vi "Actor Core.vi"(8 "error in":errorcluster, 11 "Blackstart in":refnum<class "Blackstart.lvclass">) -> (0 "error out":errorcluster, 3 "Actor out":refnum<class "Actor.lvclass">)   [LabVIEW 2018, in "Blackstart Actor.lvlib" / "Blackstart.lvclass"]
doc: "(<B>Filename</B>: Actor Framework.lvlib:Actor.lvclass:Actor Core.vi)\n\nReceives messages to the actor, reacts to them, and initiates any error handling that may shut the actor down.\n\nDescendant classes may override this VI to append parallel tasks for the actor to complete while it handles messages. Overrides use the Call Parent Method node."
uses:
  Blackstart.lvclass
  C:/Program Files (x86)/National Instruments/LabVIEW 2018/vi.lib/ActorFramework/Actor/Actor.lvclass
  C:/Users/Administrator/Desktop/LabVIEW EMS/EMS Generic Actor/EMS Generic/EMS Generic.lvclass
  C:/Users/Administrator/Desktop/LabVIEW EMS/Optimization/Startup Optimization Actor/Startup Optimization/Startup Optimization.lvclass
  C:/Users/Administrator/Desktop/LabVIEW EMS/Device Communication and Control Abstract Actor/Device Communication and Control Abstract/Device Communication and Control Abstract.lvclass
  C:/Users/Administrator/Desktop/LabVIEW EMS/Optimization/Generic Optimization Actor/Generic Optimization/Generic Optimization.lvclass
  <vilib>/ActorFramework/Actor/Actor.lvclass
  Controls/Blackstart State.ctl
  <vilib>/ORNL/CSEISMIC DDS/CSEISMIC DDS Base/Data Types/Controls/DeviceID.ctl
  <vilib>/ActorFramework/Actor/Actor.lvclass/Actor.ctl
  EMS Generic Actor/EMS Generic/EMS Generic.lvclass/EMS Generic.ctl
  <vilib>/ActorFramework/Message Enqueuer/Message Enqueuer.lvclass/Message Enqueuer.ctl
  <vilib>/ORNL/CSEISMIC DDS/CSEISMIC DDS Base/Data Types/DER_VF.ctl
  Startup Optimization Actor/Startup Optimization/Startup Optimization.lvclass/Startup Optimization.ctl
  Device Communication and Control Abstract Actor/Device Communication and Control Abstract/Device Communication and Control Abstract.lvclass/Device Communication and Control Abstract.ctl
  Device Communication and Control Abstract Actor/Device Communication and Control Abstract Messages/Set DER VF Msg/Set DER VF Msg.lvclass/Set DER VF Msg.ctl
  <vilib>/ORNL/CSEISMIC DDS/CSEISMIC DDS Base/Data Types/PCC_Transition.ctl
  Device Communication and Control Abstract Actor/Device Communication and Control Abstract Messages/Set PCC Transition Msg/Set PCC Transition Msg.lvclass/Set PCC Transition Msg.ctl
  <vilib>/ORNL/CSEISMIC DDS/CSEISMIC DDS Base/Data Types/DER_Control.ctl
  <vilib>/ORNL/CSEISMIC DDS/CSEISMIC DDS Base/Data Types/DER_setGenerationMode.ctl
  <vilib>/ORNL/CSEISMIC DDS/CSEISMIC DDS Base/Data Types/Controls/Generation Mode.ctl
  Device Communication and Control Abstract Actor/Device Communication and Control Abstract Messages/Set DER GenerationMode Msg/Set DER GenerationMode Msg.lvclass/Set DER GenerationMode Msg.ctl
  Device Communication and Control Abstract Actor/Device Communication and Control Abstract Messages/Set DER Control Msg/Set DER Control Msg.lvclass/Set DER Control Msg.ctl
  <vilib>/ORNL/CSEISMIC DDS/CSEISMIC DDS Base/Data Types/Relay_Control.ctl
  Device Communication and Control Abstract Actor/Device Communication and Control Abstract Messages/Set Relay Control Msg/Set Relay Control Msg.lvclass/Set Relay Control Msg.ctl
  <vilib>/ORNL/CSEISMIC DDS/CSEISMIC DDS Base/Data Types/Load_Control.ctl
  Device Communication and Control Abstract Actor/Device Communication and Control Abstract Messages/Set Load Control Msg/Set Load Control Msg.lvclass/Set Load Control Msg.ctl
  <vilib>/ActorFramework/Message Enqueuer/Init from Existing Queue.vi
  <vilib>/ActorFramework/Message Enqueuer/Enqueue.vi
  Device Communication and Control Abstract Actor/Device Communication and Control Abstract Messages/Set DER VF Msg/Send Set DER VF.vi
  Device Communication and Control Abstract Actor/Device Communication and Control Abstract Messages/Set PCC Transition Msg/Send Set PCC Transition.vi
  Device Communication and Control Abstract Actor/Device Communication and Control Abstract Messages/Set DER GenerationMode Msg/Send Set DER GenerationMode.vi
  Device Communication and Control Abstract Actor/Device Communication and Control Abstract Messages/Set DER Control Msg/Send Set DER Control.vi
  Device Communication and Control Abstract Actor/Device Communication and Control Abstract Messages/Set Relay Control Msg/Send Set Relay Control.vi
  Device Communication and Control Abstract Actor/Device Communication and Control Abstract Messages/Set Load Control Msg/Send Set Load Control.vi
  Device Communication and Control Abstract Actor/Device Communication and Control Abstract/Device Communication and Control Abstract.lvclass
  Device Communication and Control Abstract Actor/Device Communication and Control Abstract Messages/Set DER VF Msg/Set DER VF Msg.lvclass
  C:/Program Files (x86)/National Instruments/LabVIEW 2018/vi.lib/ActorFramework/Message/Message.lvclass
  Device Communication and Control Abstract Actor/Device Communication and Control Abstract Messages/Set PCC Transition Msg/Set PCC Transition Msg.lvclass
  Device Communication and Control Abstract Actor/Device Communication and Control Abstract Messages/Set DER GenerationMode Msg/Set DER GenerationMode Msg.lvclass
  Device Communication and Control Abstract Actor/Device Communication and Control Abstract Messages/Set DER Control Msg/Set DER Control Msg.lvclass
  Device Communication and Control Abstract Actor/Device Communication and Control Abstract Messages/Set Relay Control Msg/Set Relay Control Msg.lvclass
  Device Communication and Control Abstract Actor/Device Communication and Control Abstract Messages/Set Load Control Msg/Set Load Control Msg.lvclass
  <vilib>/ActorFramework/Stop Msg/Stop Msg.lvclass
  <vilib>/ActorFramework/Message Priority Queue/Priority Enqueue.vi
  Startup Optimization Actor/Startup Optimization/Startup Optimization.lvclass
  <vilib>/ActorFramework/Message Enqueuer/Message Enqueuer.lvclass
  <vilib>/ORNL/CSEISMIC DDS/CSEISMIC DDS Base/CSEISMIC DDS.lvclass
  Utilities/Status Messaging.llb/Status Messaging.lvlib
  EMS Generic Actor/EMS Generic/EMS Generic.lvclass
  Generic Optimization Actor/Generic Optimization/Generic Optimization.lvclass
panel:
  out "Devices":string[](array[string])
  in  "Ignore missing devices?":bool
  out "Status":T1
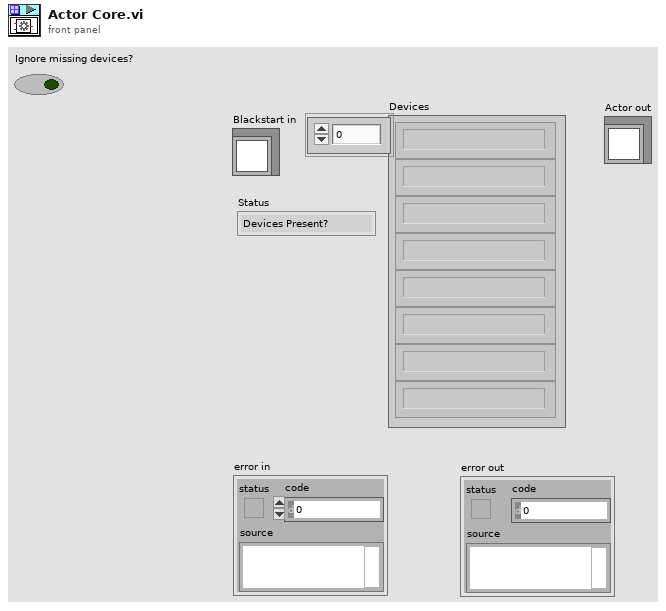
[diagram p1: front panel]
types:
  T1 = typedef "Blackstart Actor.lvlib/Blackstart.lvclass/Blackstart State.ctl" = enum16{"Devices Present?", "Group Devices", "Set VF Device", "Island", "Activate VF Device", "Close Relays", "Activate Loads", "Activate DERs", "Success", "Failure"}
  T2 = typedef "CSEISMIC DDS.lvlib/CSEISMIC DDS.lvclass/DeviceID.ctl" = string
  T3 = enum32{"Invalid", "Standard", "Closed", "Hidden", "Minimized", "Maximized"}
  T4 = typedef "CSEISMIC DDS.lvlib/CSEISMIC DDS.lvclass/DER_VF.ctl" = cluster{"DeviceID":T2}
  T5 = typedef "CSEISMIC DDS.lvlib/CSEISMIC DDS.lvclass/DER_setGenerationMode.ctl" = cluster{"DeviceID":T2, "Mode":T6}
  T6 = typedef "CSEISMIC DDS.lvlib/CSEISMIC DDS.lvclass/Generation Mode.ctl" = enum32{"Invalid", "PQ", "Droop", "PV", "PF", "VF"}
  T7 = typedef "CSEISMIC DDS.lvlib/CSEISMIC DDS.lvclass/DER_Control.ctl" = cluster{"DeviceID":T2, "Activate":bool, "Deactivate":bool}
  T8 = typedef "EMS Generic Actor.lvlib/EMS Generic.lvclass/Global Configuration.ctl" = cluster{"Microgrid ID":u8, "VF Device ID":T2, "Ongrid VF Priority":T2[], "Offgrid VF Priority":T2[], "AutoSwap Offgrid VF":u32, "AutoSwap Offgrid VF Delay (sec)":dbl, "AutoSwap Resynch VF":u32, "PCC Device ID":T2, "Device ID Array":T2[], "Nominal Voltage":dbl, "Nominal Frequency":dbl, "Resynch Timeout (sec)":dbl, "Island VF Activate Timeout (sec)":dbl, "Island PCC Target Power (kW)":dbl, "Island PCC Target Power Timeout (sec)":dbl, "Island Grid Settle Time (sec)":dbl, "Island PCC Failure Timeout (sec)":dbl, "Activation Devices Present Timeout (sec)":dbl, "Activation Devices Activated Timeout (sec)":dbl, "Blackstart VF GenMode Wait (sec)":dbl, "Blackstart VF DERCtrl Wait (sec)":dbl, "Blackstart Success Wait (sec)":dbl, "OnGrid Optimization Delay (sec)":dbl, "OffGrid Optimization Delay (sec)":dbl, "Resynch Frequency (Hz)":dbl, "Optimization Path":string}
  T9 = typedef "CSEISMIC DDS.lvlib/CSEISMIC DDS.lvclass/PCC_Transition.ctl" = cluster{"DeviceID":T2, "Island":bool, "Resynchronize":bool}
  T10 = typedef "CSEISMIC DDS.lvlib/CSEISMIC DDS.lvclass/IED_Status.ctl" = cluster{"DeviceID":T2, "Timestamp":T11, "MicrogridID":u8, "Active":bool, "Inactive":bool, "Error":i32, "Fault":bool, "ErrorString":string}
  T11 = typedef "CSEISMIC DDS.lvlib/CSEISMIC DDS.lvclass/Timestamp.ctl" = cluster{"Seconds":u64, "Remainder":u64}
  T12 = typedef "CSEISMIC DDS.lvlib/CSEISMIC DDS.lvclass/Relay_Control.ctl" = cluster{"DeviceID":T2, "Activate":bool, "Deactivate":bool}
  T13 = typedef "CSEISMIC DDS.lvlib/CSEISMIC DDS.lvclass/Load_Control.ctl" = cluster{"DeviceID":T2, "Activate":bool, "Deactivate":bool}
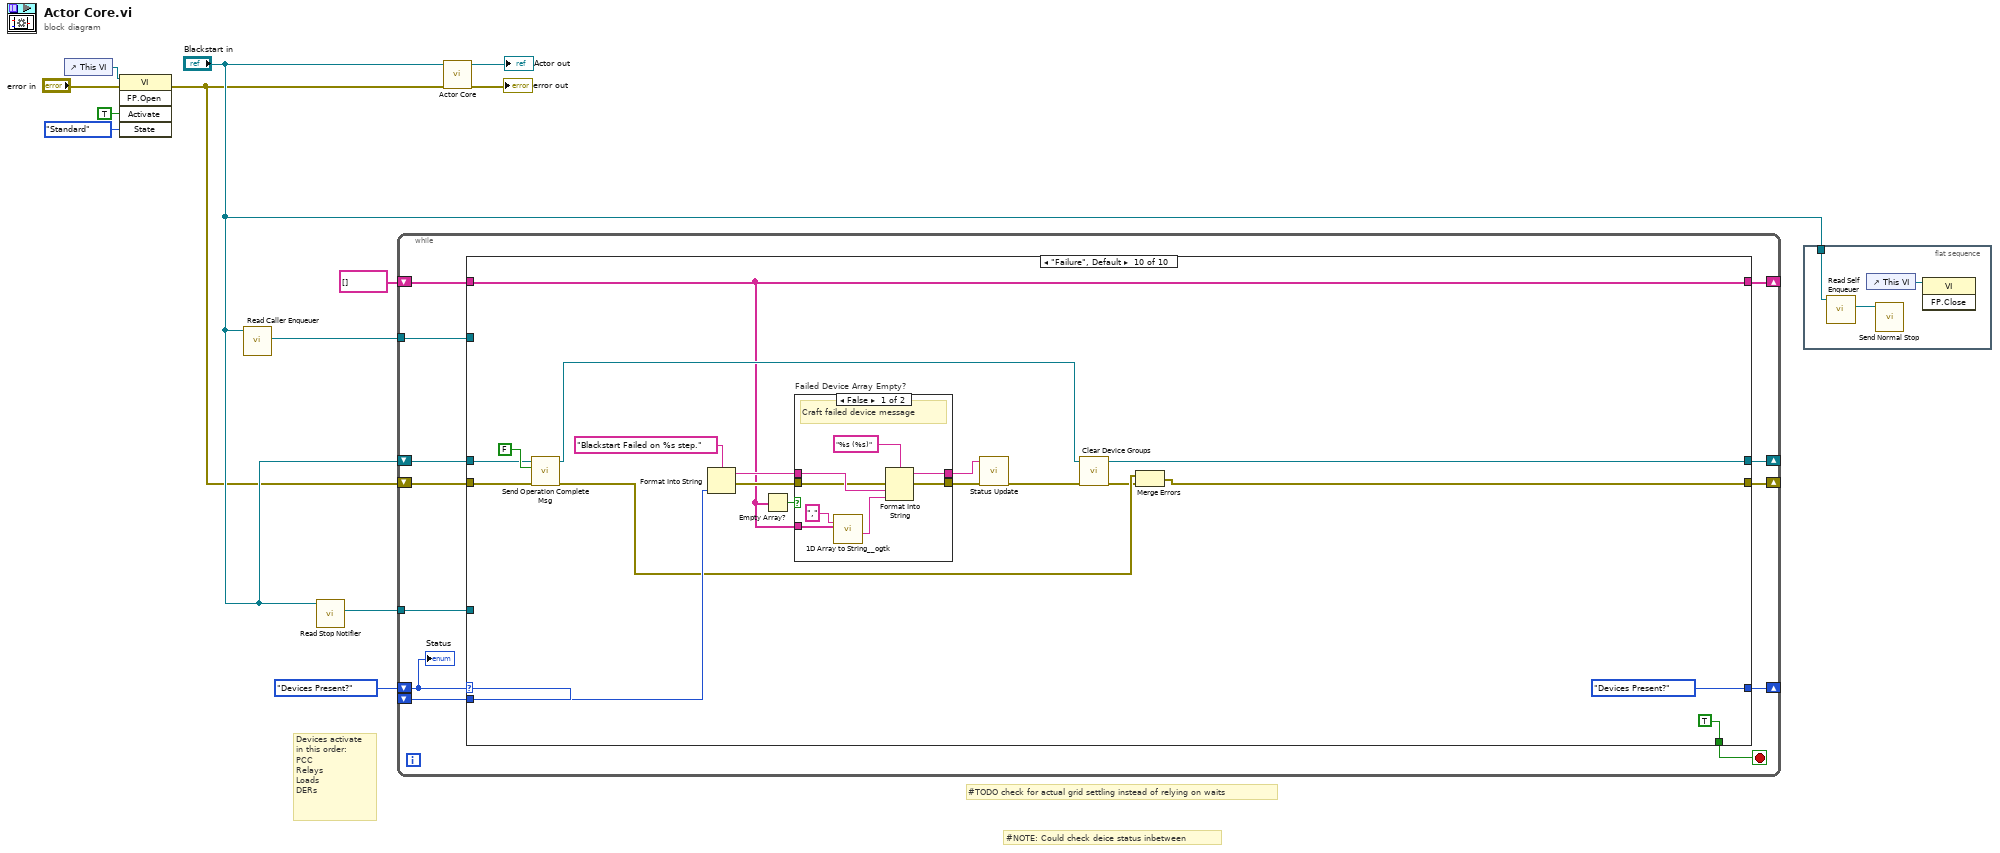
[diagram p0: block diagram]
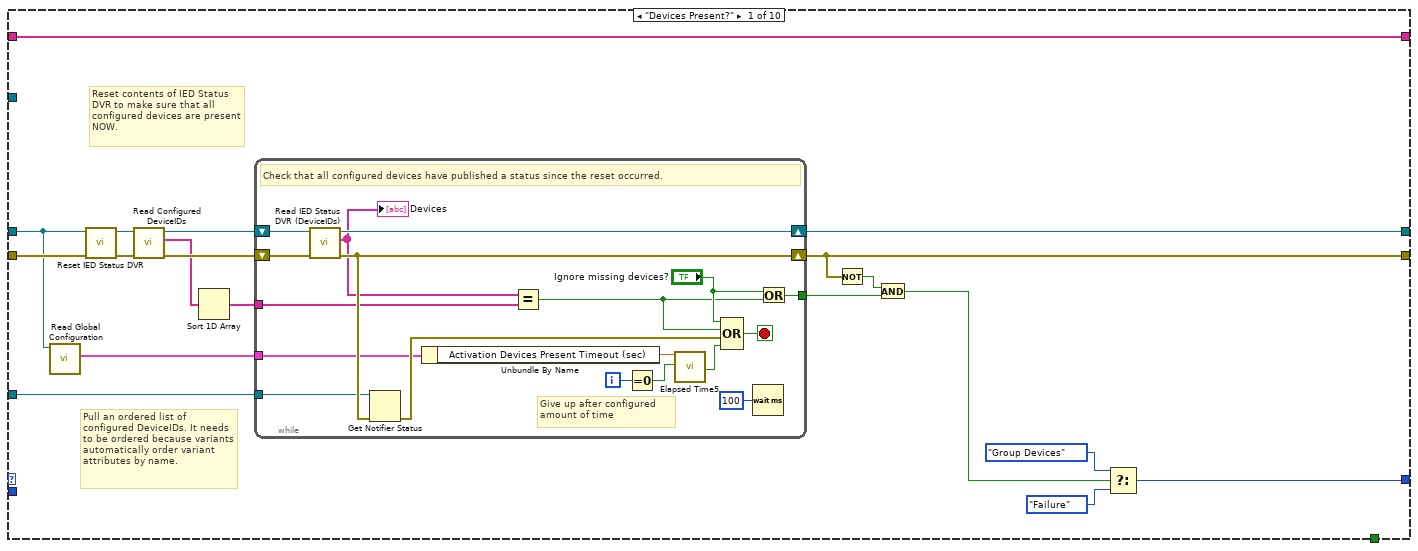
[diagram p2: hidden frame]
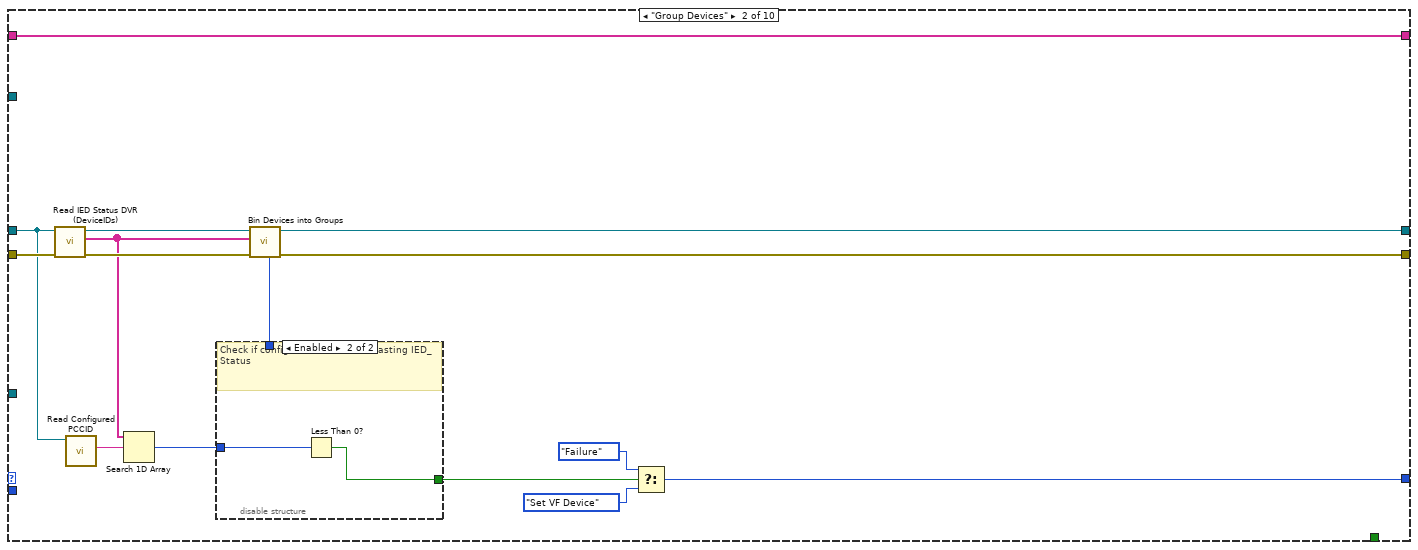
[diagram p3: hidden frame]
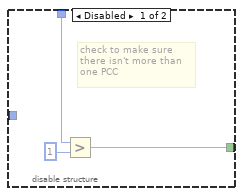
[diagram p4: hidden frame]
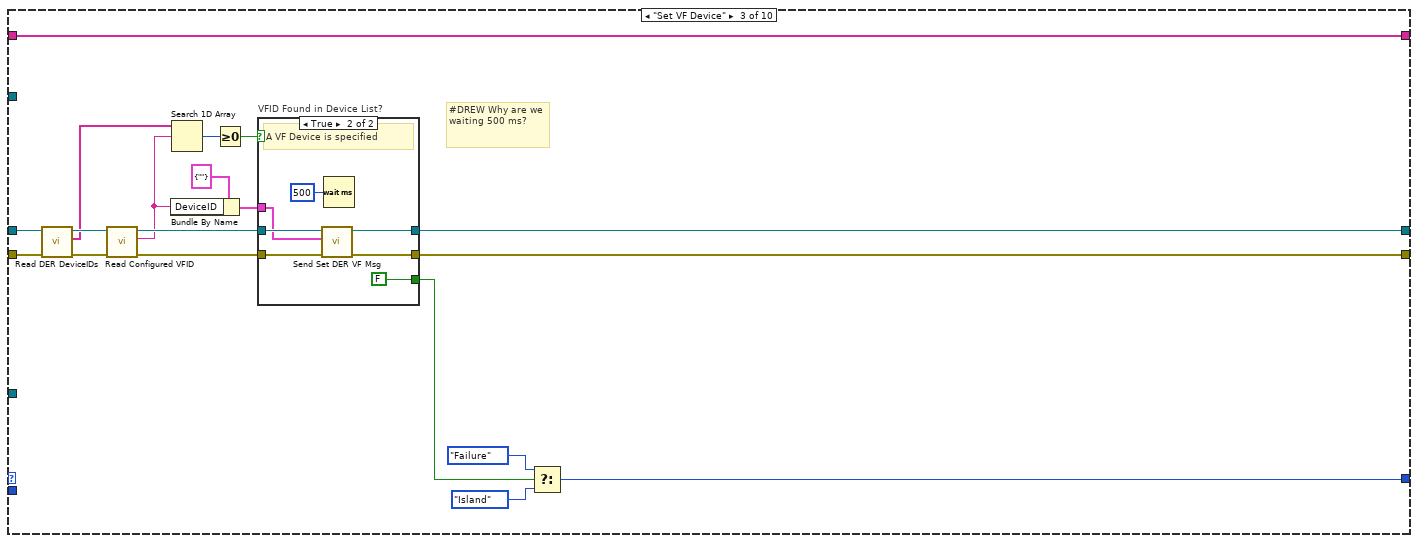
[diagram p5: hidden frame]
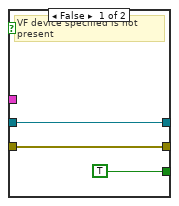
[diagram p6: hidden frame]
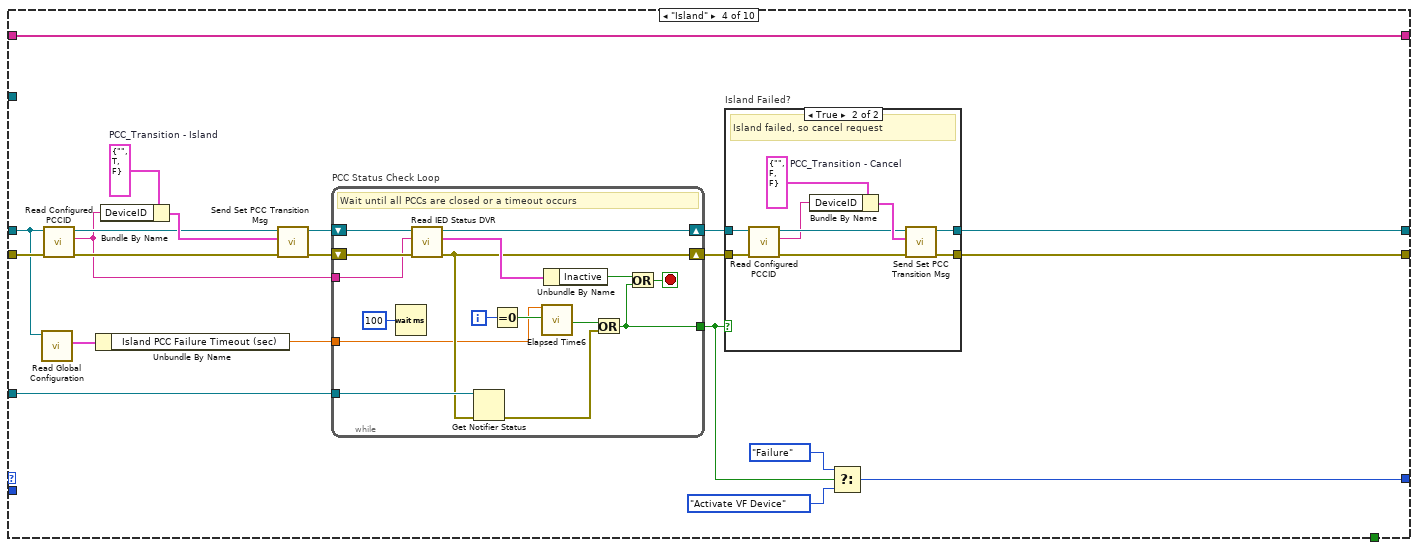
[diagram p7: hidden frame]
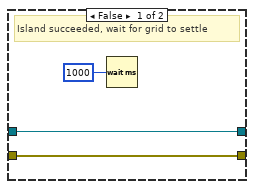
[diagram p8: hidden frame]
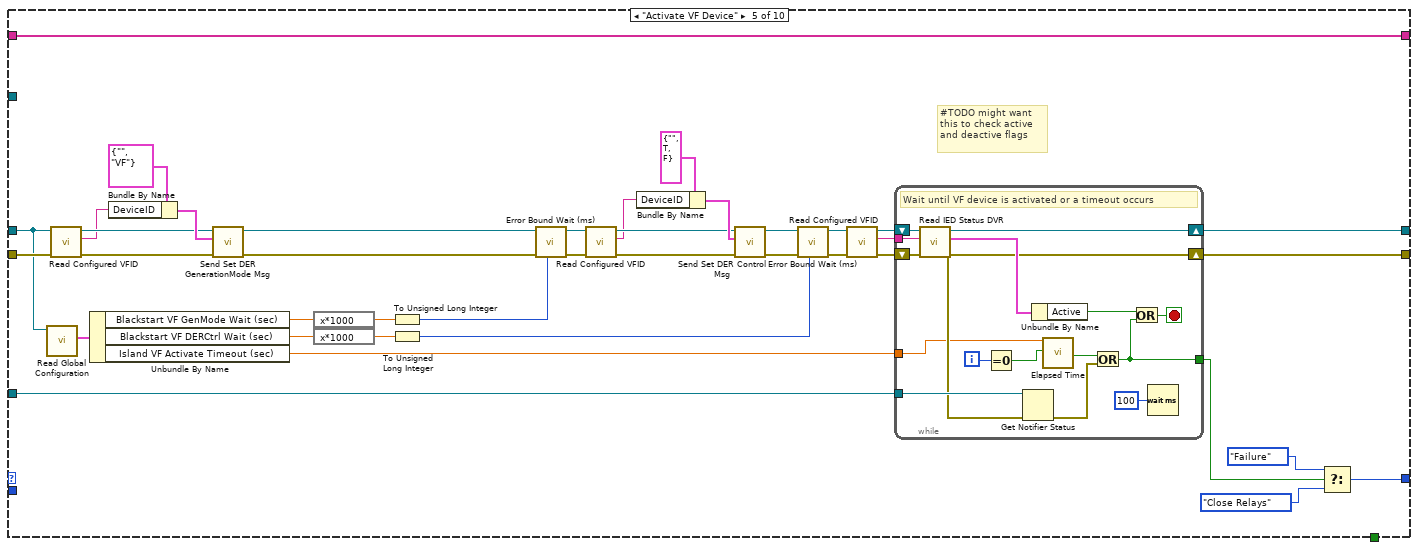
[diagram p9: hidden frame]
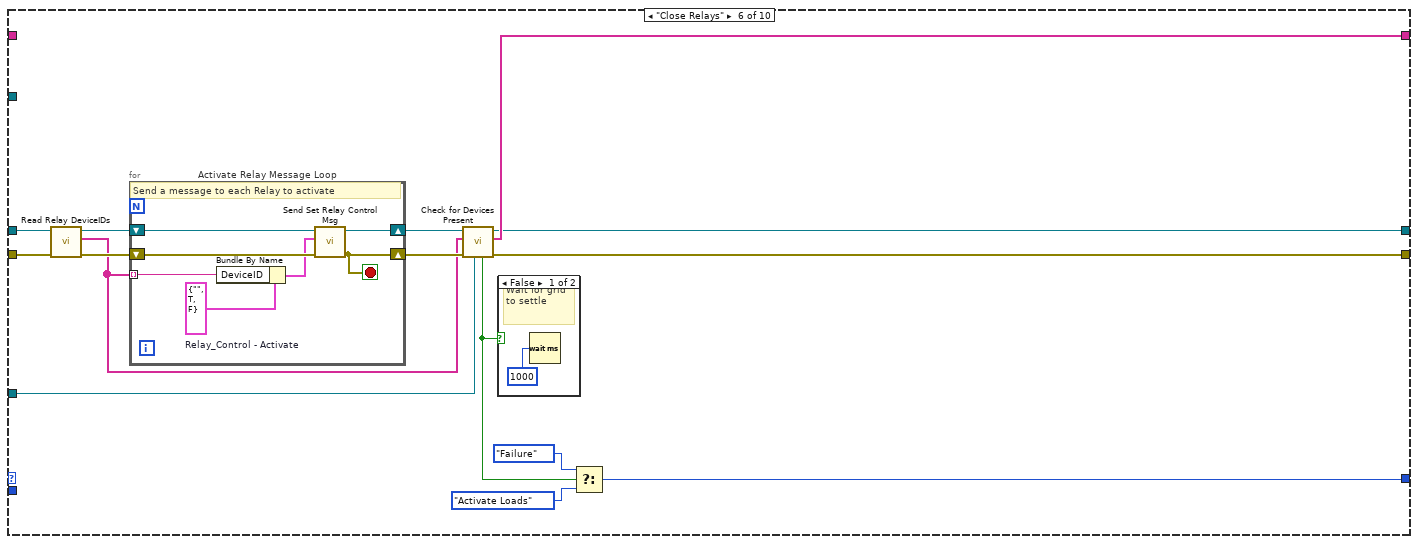
[diagram p10: hidden frame]
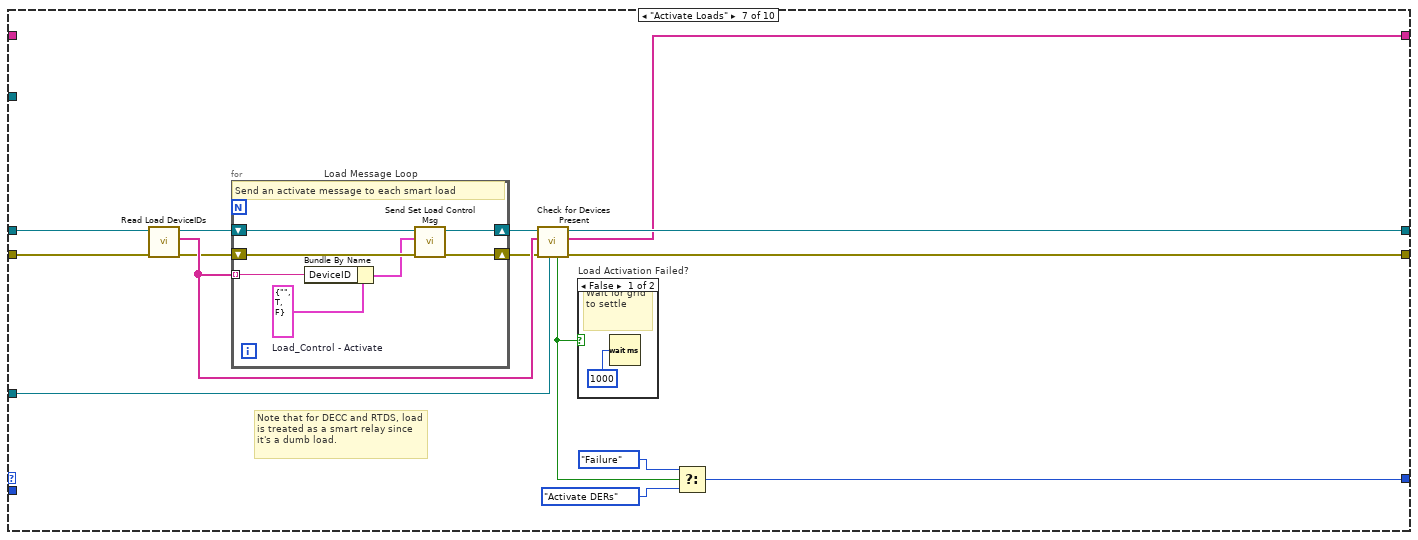
[diagram p12: hidden frame]
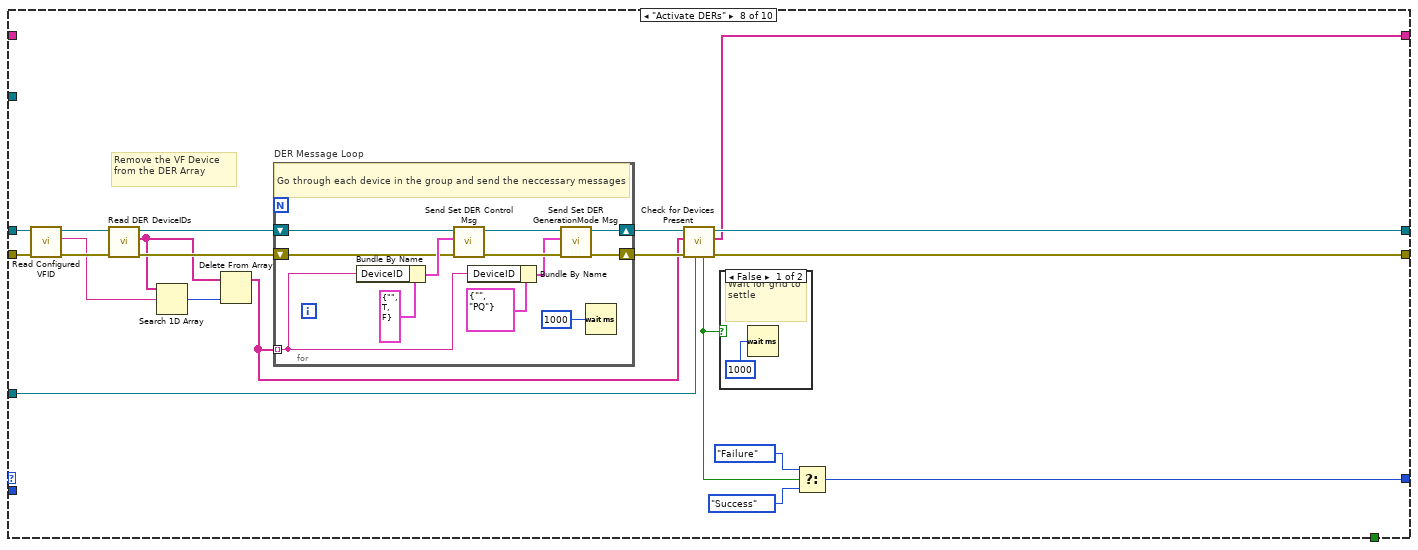
[diagram p14: hidden frame]
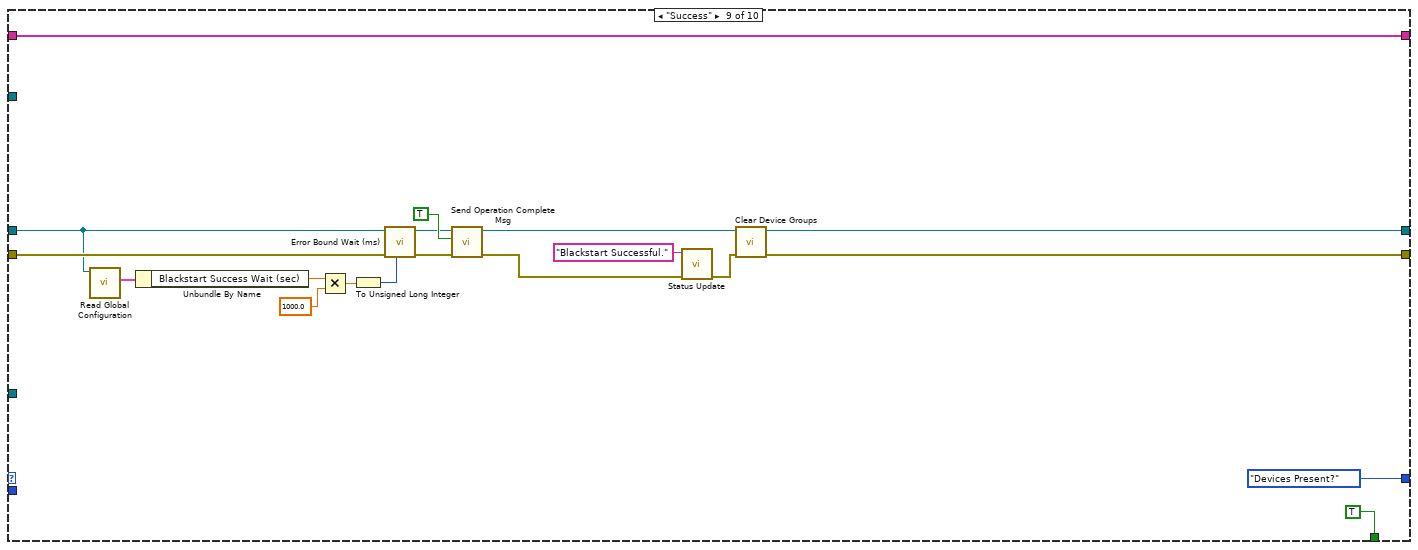
[diagram p16: hidden frame]
diagram:
  w2 = Blackstart_State."Devices Present?"
  # "#TODO check for actual grid settling instead of relying on waits"
  # "Devices activate in this order:\nPCC\nRelays\nLoads\nDERs"
  # "#NOTE: Could check deice status inbetween"
  n1 = control-ref of="This VI"() -> (w7:refnum<vi>)
  n2 = invoke class="VI" method="FP.Open"(reference=w7, error in="error in", "Activate"=TRUE ("Activate?"), "State"=T3."Standard") -> (error out=w4:errorcluster)  [unwired: 1 in, 4 out]
  n3 = call <vilib>:"Read Caller Enqueuer.vi"("Actor"="Blackstart in") -> ("Caller Enqueuer"=w10:refnum<class "Message Enqueuer.lvclass">)  [unwired: 10 in]
  n4 = call "Read Stop Notifier.vi"("EMS Generic in"="Blackstart in") -> ("stop"=w1:refnum<notifier>)  [unwired: 9 in, 1 out]
  n5 = while {
    shift-right: [w23] -> _
    shift-left: w2 -> [w24]
    tunnel: w10 -> [w22]
    shift-left: w2 -> [w19]
    tunnel: w1 -> [w18]
    shift-right: [w17] -> _
    shift-left: T2[] [] -> [w16]
    shift-right: [w14] -> _
    shift-left: "Blackstart in" -> [w21]
    shift-right: [w13] -> _
    shift-left: w4 -> [w15]
    stop <- w20 stop-if-true
    n6 = case shown="\"Failure\", Default" w24 {
      tunnel: [w42 w76 w98 w118 w195 w225 w248 w276 Blackstart_State."Devices Present?" Blackstart_State."Devices Present?"] -> w23
      tunnel: w22 -> [_ _ _ _ _ _ _ _ _ _]
      tunnel: w21 -> [w26 w64 w88 w113 w168 w224 w242 w268 w297 w317]
      tunnel: [_ _ _ _ _ _ _ _ TRUE TRUE] -> w20
      tunnel: w19 -> [_ _ _ _ _ _ _ _ _ w313]
      tunnel: w18 -> [w31 _ _ w124 w192 w218 w240 w264 _ _]
      tunnel: [w40 w75 w97 w131 w193 w216 w236 w261 w307 w314] -> w17
      tunnel: w16 -> [w40 w75 w97 w131 w193 _ _ _ w307 w314]
      tunnel: w15 -> [w30 w72 w86 w116 w186 w223 w241 w269 w306 w316]
      tunnel: [w29 w69 w90 w123 w170 w215 w239 w262 w301 w315] -> w14
      tunnel: [w28 w67 w91 w122 w169 w214 w238 w259 w300 w310] -> w13
      frame "Devices Present?" {
        # "Pull an ordered list of configured DeviceIDs. It needs to be ordered because variants automatically order variant attributes by name."
        # "Reset contents of IED Status DVR to make sure that all configured devices are present NOW."
        n7 = call "Read Global Configuration.vi"("EMS Generic in"=w26) -> ("Global Configuration"=w25:T8)  [unwired: 8 in, 2 out]
        n8 = call "Reset IED Status DVR.vi"("error in"=w30, "SCADA in"=w26) -> ("error out"=w38:errorcluster, "dup SCADA out"=w37:refnum<class "Blackstart.lvclass">)  [unwired: 8 in]
        n9 = call "Read Configured DeviceIDs.vi"("error in"=w38, "EMS Generic in"=w37) -> ("error out"=w34:errorcluster, "DeviceIDs"=w32:T2[], "EMS Generic out"=w39:refnum<class "Blackstart.lvclass">)  [unwired: 7 in]
        n10 = Sort 1D Array(array=w32) -> (sorted array=w33:T2[])
        n11 = while {
          tunnel: w33 -> [w59]
          shift-right: [w61] -> w28
          shift-left: w34 -> [w49]
          tunnel: [w54] -> w35
          tunnel: w31 -> [w58]
          shift-right: [w47] -> w29
          shift-left: w39 -> [w48]
          tunnel: w25 -> [w45]
          i -> [w51]
          stop <- w53 stop-if-true
          # "Give up after configured amount of time"
          # "Check that all configured devices have published a status since the reset occurred."
          n12 = call "Read IED Status DVR (DeviceIDs).vi"("error in"=w49, "EMS Generic in"=w48) -> ("error out"=w61:errorcluster, "DeviceID Array"=w46:T2[], "EMS Generic out"=w47:refnum<class "Blackstart.lvclass">)  [unwired: 7 in]
          "Devices" <- w46
          n13 = Get Notifier Status(notifier=w58, error in (no error)=w61) -> (error out=w57:errorcluster)  [unwired: 4 out]
          n14 = Unbundle By Name(w45) -> ("Activation Devices Present Timeout (sec)"=w44:dbl)
          n15 = Equal?(x=w46, y=w59) -> (x = y?=w55:bool)
          n16 = Equal To 0?(x=w51) -> (x = 0?=w50:bool)
          n17 = call "Elapsed Time5"("Time Target (s)"=w44, "Reset"=w50) -> ("Time has Elapsed"=w52:bool)  [unwired: 10 in, 7 out]
          n18 = Compound Arithmetic op=OR("Ignore missing devices?", w55, w57, w52) -> (w53:bool)
          n19 = Wait (ms)(milliseconds to wait=u32 100) -> ()  [unwired: 1 out]
          n20 = Or(x="Ignore missing devices?", y=w55) -> (x .or. y?=w54:bool)
        }
        n21 = Not(x=w28) -> (.not. x?=w36:bool)
        n22 = And(x=w36, y=w35) -> (x .and. y?=w27:bool)
        n23 = Select(t=Blackstart_State."Group Devices", s=w27, f=Blackstart_State."Failure") -> (s? t:f=w42:T1)
      }
      frame "Group Devices" {
        n24 = call "Read IED Status DVR (DeviceIDs).vi"("error in"=w72, "EMS Generic in"=w64) -> ("error out"=w68:errorcluster, "DeviceID Array"=w63:T2[], "EMS Generic out"=w70:refnum<class "Blackstart.lvclass">)  [unwired: 7 in]
        n25 = call "Read Configured PCCID.vi"("EMS Generic in"=w64) -> ("PCCID"=w65:T2)  [unwired: 8 in, 2 out]
        n26 = Search 1D Array(1D array=w63, element=w65) -> (index of element=w62:i32)  [unwired: 1 in]
        n27 = call "Bin Devices into Groups.vi"("error in (no error)"=w68, "DeviceID Array"=w63, "Startup Optimization in"=w70) -> ("error out"=w67:errorcluster, "Startup Optimization out"=w69:refnum<class "Blackstart.lvclass">, "Number of PCCs"=w66:i16)  [unwired: 6 in]
        n28 = disable-structure shown="Enabled" {
          disable-tunnel: [w78 w80] -> w71
          disable-tunnel: w66 -> [w77 _]
          disable-tunnel: w62 -> [_ w81]
          frame Disabled {
            # "check to make sure there isn't more than one PCC"
            n29 = Greater?(x=w77, y=i16 1) -> (0:w78:bool)
          }
          frame Enabled {
            # "Check if configured PCC is broadcasting IED_Status"
            n30 = Less Than 0?(x=w81) -> (x < 0?=w80:bool)
          }
        }
        n31 = Select(t=Blackstart_State."Failure", s=w71, f=Blackstart_State."Set VF Device") -> (s? t:f=w76:T1)
      }
      frame "Set VF Device" {
        # "#DREW Why are we waiting 500 ms?"
        n32 = call "Read DER DeviceIDs.vi"("error in"=w86, "Startup Optimization in"=w88) -> ("error out"=w85:errorcluster, "DERs"=w84:T2[], "Startup Optimization out"=w87:refnum<class "Blackstart.lvclass">)  [unwired: 7 in]
        n33 = call "Read Configured VFID.vi"("error in"=w85, "EMS Generic in"=w87) -> ("error out"=w96:errorcluster, "VFID"=w94:T2, "EMS Generic out"=w95:refnum<class "Blackstart.lvclass">)  [unwired: 7 in]
        n34 = Bundle By Name(cluster=T4 {"DeviceID"=""} ("DER_VF"), "DeviceID"=w94) -> (w93:T4)
        n35 = Search 1D Array(1D array=w84, element=w94) -> (index of element=w83:i32)  [unwired: 1 in]
        n36 = Greater Or Equal To 0?(x=w83) -> (x >= 0?=w82:bool)
        n37 = case "VFID Found in Device List?" shown="True" w82 {
          tunnel: [TRUE FALSE] -> w89
          tunnel: w93 -> [_ w107]
          tunnel: w95 -> [w102 w108]
          tunnel: [w102 w106] -> w90
          tunnel: w96 -> [w101 w105]
          tunnel: [w101 w104] -> w91
          frame False {
            # "VF device specified is not present"
          }
          frame True {
            # "A VF Device is specified"
            n38 = call "Send Set DER VF Msg.vi"("error in"=w105, "DER_VF"=w107, "SCADA Sub Abstract in"=w108) -> ("error out"=w104:errorcluster, "dup SCADA Sub Abstract"=w106:refnum<class "Blackstart.lvclass">)  [unwired: 7 in]
            n39 = Wait (ms)(milliseconds to wait=u32 500) -> ()  [unwired: 1 out]
          }
        }
        n40 = Select(t=Blackstart_State."Failure", s=w89, f=Blackstart_State."Island") -> (s? t:f=w98:T1)
      }
      frame "Island" {
        w125 = T9 {"DeviceID"="", "Island"=TRUE, "Resynchronize"=FALSE}  # PCC_Transition - Island
        n41 = call "Read Global Configuration.vi"("EMS Generic in"=w113) -> ("Global Configuration"=w117:T8)  [unwired: 8 in, 2 out]
        n42 = call "Read Configured PCCID.vi"("error in"=w116, "EMS Generic in"=w113) -> ("error out"=w114:errorcluster, "PCCID"=w111:T2, "EMS Generic out"=w115:refnum<class "Blackstart.lvclass">)  [unwired: 7 in]
        n43 = Unbundle By Name(w117) -> ("Island PCC Failure Timeout (sec)"=w112:dbl)
        n44 = Bundle By Name(cluster=w125, "DeviceID"=w111) -> (w130:T9)
        n45 = call "Send Set PCC Transition Msg.vi"("error in"=w114, "PCC_Transition"=w130, "SCADA Sub Abstract in"=w115) -> ("error out"=w128:errorcluster, "dup SCADA Sub Abstract"=w129:refnum<class "Blackstart.lvclass">)  [unwired: 7 in]
        n46 = while "PCC Status Check Loop" {
          tunnel: [w157] -> w119
          tunnel: w124 -> [w156]
          shift-right: [w148] -> w126
          shift-left: w128 -> [w145]
          shift-right: [w149] -> w127
          shift-left: w129 -> [w146]
          tunnel: w112 -> [w147]
          tunnel: w111 -> [w144]
          i -> [w155]
          stop <- w158 stop-if-true
          # "Wait until all PCCs are closed or a timeout occurs"
          n47 = Wait (ms)(milliseconds to wait=u32 100) -> ()  [unwired: 1 out]
          n48 = call "Read IED Status DVR.vi"("error in"=w145, "DeviceID"=w144, "EMS Generic in"=w146) -> ("error out"=w148:errorcluster, "IED_Status"=w152:T10, "EMS Generic out"=w149:refnum<class "Blackstart.lvclass">)  [unwired: 5 in, 1 out]
          n49 = Get Notifier Status(notifier=w156, error in (no error)=w148) -> (error out=w150:errorcluster)  [unwired: 4 out]
          n50 = Equal To 0?(x=w155) -> (x = 0?=w154:bool)
          n51 = call "Elapsed Time6"("Time Target (s)"=w147, "Reset"=w154) -> ("Time has Elapsed"=w151:bool)  [unwired: 10 in, 7 out]
          n52 = Unbundle By Name(w152) -> ("Inactive"=w159:bool)
          n53 = Or(x=w151, y=w150) -> (x .or. y?=w157:bool)
          n54 = Or(x=w159, y=w157) -> (x .or. y?=w158:bool)
        }
        n55 = case "Island Failed?" shown="True" w119 {
          tunnel: w127 -> [w134 w139]
          tunnel: [w134 w141] -> w123
          tunnel: w126 -> [w133 w138]
          tunnel: [w133 w142] -> w122
          frame False {
            # "Island succeeded, wait for grid to settle"
            n56 = Wait (ms)(milliseconds to wait=u32 1000) -> ()  [unwired: 1 out]
          }
          frame True {
            w143 = T9 {"DeviceID"="", "Island"=FALSE, "Resynchronize"=FALSE}  # PCC_Transition - Cancel
            # "Island failed, so cancel request"
            n57 = call "Read Configured PCCID.vi"("error in"=w138, "EMS Generic in"=w139) -> ("error out"=w137:errorcluster, "PCCID"=w135:T2, "EMS Generic out"=w136:refnum<class "Blackstart.lvclass">)  [unwired: 7 in]
            n58 = Bundle By Name(cluster=w143, "DeviceID"=w135) -> (w140:T9)
            n59 = call "Send Set PCC Transition Msg.vi"("error in"=w137, "PCC_Transition"=w140, "SCADA Sub Abstract in"=w136) -> ("error out"=w142:errorcluster, "dup SCADA Sub Abstract"=w141:refnum<class "Blackstart.lvclass">)  [unwired: 7 in]
          }
        }
        n60 = Select(t=Blackstart_State."Failure", s=w119, f=Blackstart_State."Activate VF Device") -> (s? t:f=w118:T1)
      }
      frame "Activate VF Device" {
        # "#TODO might want this to check active and deactive flags"
        n61 = call "Read Global Configuration.vi"("EMS Generic in"=w168) -> ("Global Configuration"=w167:T8)  [unwired: 8 in, 2 out]
        n62 = call "Read Configured VFID.vi"("error in"=w186, "EMS Generic in"=w168) -> ("error out"=w184:errorcluster, "VFID"=w172:T2, "EMS Generic out"=w185:refnum<class "Blackstart.lvclass">)  [unwired: 7 in]
        n63 = Unbundle By Name(w167) -> ("Blackstart VF GenMode Wait (sec)"=w166:dbl, "Blackstart VF DERCtrl Wait (sec)"=w162:dbl, "Island VF Activate Timeout (sec)"=w160:dbl)
        n64 = Bundle By Name(cluster=T5 {"DeviceID"="", "Mode"=enum."VF"} ("DER_setGenerationMode"), "DeviceID"=w172) -> (w187:T5)
        n65 = call "Send Set DER GenerationMode Msg.vi"("error in"=w184, "DER_setGenerationMode"=w187, "SCADA Sub Abstract in"=w185) -> ("error out"=w183:errorcluster, "SCADA Sub Abstract out"=w181:refnum<class "Blackstart.lvclass">)  [unwired: 7 in]
        n66 = expression code="x*1000"(w166) -> (w165:dbl)
        n67 = expression code="x*1000"(w162) -> (w163:dbl)
        n68 = To Unsigned Long Integer(number=w165) -> (unsigned 32bit integer=w164:u32)
        n69 = To Unsigned Long Integer(number=w163) -> (unsigned 32bit integer=w161:u32)
        n70 = call "Error Bound Wait (ms).vi"("milliseconds to wait (100)"=w164, "error in"=w183) -> ("error out"=w182:errorcluster)  [unwired: 9 in]
        n71 = call "Read Configured VFID.vi"("error in"=w182, "EMS Generic in"=w181) -> ("error out"=w179:errorcluster, "VFID"=w178:T2, "EMS Generic out"=w180:refnum<class "Blackstart.lvclass">)  [unwired: 7 in]
        n72 = Bundle By Name(cluster=T7 {"DeviceID"="", "Activate"=TRUE, "Deactivate"=FALSE} ("DER_Control"), "DeviceID"=w178) -> (w188:T7)
        n73 = call "Send Set DER Control Msg.vi"("error in"=w179, "DER_Control"=w188, "SCADA Sub Abstract in"=w180) -> ("error out"=w177:errorcluster, "dup SCADA Sub Abstract"=w174:refnum<class "Blackstart.lvclass">)  [unwired: 7 in]
        n74 = call "Error Bound Wait (ms).vi"("milliseconds to wait (100)"=w161, "error in"=w177) -> ("error out"=w176:errorcluster)  [unwired: 9 in]
        n75 = call "Read Configured VFID.vi"("error in"=w176, "EMS Generic in"=w174) -> ("error out"=w175:errorcluster, "VFID"=w171:T2, "EMS Generic out"=w173:refnum<class "Blackstart.lvclass">)  [unwired: 7 in]
        n76 = while {
          tunnel: w171 -> [w202]
          tunnel: [w209] -> w189
          tunnel: w192 -> [w208]
          shift-right: [w199] -> w170
          shift-left: w173 -> [w203]
          shift-right: [w198] -> w169
          shift-left: w175 -> [w201]
          tunnel: w160 -> [w197]
          i -> [w206]
          stop <- w211 stop-if-true
          # "Wait until VF device is activated or a timeout occurs"
          n77 = call "Read IED Status DVR.vi"("error in"=w201, "DeviceID"=w202, "EMS Generic in"=w203) -> ("error out"=w198:errorcluster, "IED_Status"=w200:T10, "EMS Generic out"=w199:refnum<class "Blackstart.lvclass">)  [unwired: 5 in, 1 out]
          n78 = Equal To 0?(x=w206) -> (x = 0?=w205:bool)
          n79 = Get Notifier Status(notifier=w208, error in (no error)=w198) -> (error out=w207:errorcluster)  [unwired: 4 out]
          n80 = Unbundle By Name(w200) -> ("Active"=w212:bool)
          n81 = call "Elapsed Time"("Time Target (s)"=w197, "Reset"=w205) -> ("Time has Elapsed"=w210:bool)  [unwired: 10 in, 7 out]
          n82 = Or(x=w210, y=w207) -> (x .or. y?=w209:bool)
          n83 = Or(x=w212, y=w209) -> (x .or. y?=w211:bool)
          n84 = Wait (ms)(milliseconds to wait=u32 100) -> ()  [unwired: 1 out]
        }
        n85 = Select(t=Blackstart_State."Failure", s=w189, f=Blackstart_State."Close Relays") -> (s? t:f=w195:T1)
      }
      frame "Close Relays" {
        n86 = call "Read Relay DeviceIDs.vi"("error in (no error)"=w223, "Startup Optimization in"=w224) -> ("error out"=w221:errorcluster, "Relays"=w217:T2[], "Startup Optimization out"=w222:refnum<class "Blackstart.lvclass">)  [unwired: 7 in]
        n87 = for "Activate Relay Message Loop" {
          tunnel: w217 -> [w233] mode=indexing
          shift-right: [w230] -> w219
          shift-left: w221 -> [w229]
          shift-right: [w231] -> w220
          shift-left: w222 -> [w232]
          stop <- w230 stop-if-true
          w234 = T12 {"DeviceID"="", "Activate"=TRUE, "Deactivate"=FALSE}  # Relay_Control - Activate
          # "Send a message to each Relay to activate"
          n88 = Bundle By Name(cluster=w234, "DeviceID"=w233) -> (w228:T12)
          n89 = call "Send Set Relay Control Msg.vi"("error in"=w229, "Relay_Control"=w228, "SCADA Sub Abstract in"=w232) -> ("error out"=w230:errorcluster, "dup SCADA Sub Abstract"=w231:refnum<class "Blackstart.lvclass">)  [unwired: 7 in]
        }
        n90 = call "Check for Devices Present.vi"("stop notifier reference"=w218, "error in"=w219, "Devices in"=w217, "Startup Optimization in"=w220) -> ("error out"=w214:errorcluster, "Failed Devices"=w216:T2[], "Startup Optimization out"=w215:refnum<class "Blackstart.lvclass">, "Time has Elapsed"=w213:bool)  [unwired: 4 in]
        n91 = case shown="False" w213 {
          frame False {
            # "Wait for grid to settle"
            n92 = Wait (ms)(milliseconds to wait=u32 1000) -> ()  [unwired: 1 out]
          }
          frame True {
          }
        }
        n93 = Select(t=Blackstart_State."Failure", s=w213, f=Blackstart_State."Activate Loads") -> (s? t:f=w225:T1)
      }
      frame "Activate Loads" {
        # "Note that for DECC and RTDS, load is treated as a smart relay since it's a dumb load."
        n94 = call "Read Load DeviceIDs.vi"("error in (no error)"=w241, "Startup Optimization in"=w242) -> ("error out"=w246:errorcluster, "Loads"=w247:T2[], "Startup Optimization out"=w245:refnum<class "Blackstart.lvclass">)  [unwired: 7 in]
        n95 = for "Load Message Loop" {
          tunnel: w247 -> [w258] mode=indexing
          shift-right: [w254] -> w243
          shift-left: w246 -> [w253]
          shift-right: [w255] -> w244
          shift-left: w245 -> [w256]
          w257 = T13 {"DeviceID"="", "Activate"=TRUE, "Deactivate"=FALSE}  # Load_Control - Activate
          # "Send an activate message to each smart load"
          n96 = Bundle By Name(cluster=w257, "DeviceID"=w258) -> (w252:T13)
          n97 = call "Send Set Load Control Msg.vi"("error in"=w253, "Load_Control"=w252, "SCADA Sub Abstract in"=w256) -> ("error out"=w254:errorcluster, "dup SCADA Sub Abstract"=w255:refnum<class "Blackstart.lvclass">)  [unwired: 7 in]
        }
        n98 = call "Check for Devices Present.vi"("stop notifier reference"=w240, "error in"=w243, "Devices in"=w247, "Startup Optimization in"=w244) -> ("error out"=w238:errorcluster, "Failed Devices"=w236:T2[], "Startup Optimization out"=w239:refnum<class "Blackstart.lvclass">, "Time has Elapsed"=w237:bool)  [unwired: 4 in]
        n99 = case "Load Activation Failed?" shown="False" w237 {
          frame False {
            # "Wait for grid to settle"
            n100 = Wait (ms)(milliseconds to wait=u32 1000) -> ()  [unwired: 1 out]
          }
          frame True {
          }
        }
        n101 = Select(t=Blackstart_State."Failure", s=w237, f=Blackstart_State."Activate DERs") -> (s? t:f=w248:T1)
      }
      frame "Activate DERs" {
        # "Remove the VF Device from the DER Array"
        n102 = call "Read Configured VFID.vi"("error in"=w269, "EMS Generic in"=w268) -> ("error out"=w278:errorcluster, "VFID"=w271:T2, "EMS Generic out"=w270:refnum<class "Blackstart.lvclass">)  [unwired: 7 in]
        n103 = call "Read DER DeviceIDs.vi"("error in"=w278, "Startup Optimization in"=w270) -> ("error out"=w277:errorcluster, "DERs"=w272:T2[], "Startup Optimization out"=w267:refnum<class "Blackstart.lvclass">)  [unwired: 7 in]
        n104 = Search 1D Array(1D array=w272, element=w271) -> (index of element=w273:i32)  [unwired: 1 in]
        n105 = Delete From Array(array=w272, index=w273) -> (array with subset deleted=w263:T2[])  [unwired: 1 in, 1 out]
        n106 = for "DER Message Loop" {
          tunnel: w263 -> [w288] mode=indexing
          shift-right: [w281] -> w265
          shift-left: w277 -> [w284]
          shift-right: [w282] -> w266
          shift-left: w267 -> [w286]
          # "Go through each device in the group and send the neccessary messages"
          n107 = Bundle By Name(cluster=T7 {"DeviceID"="", "Activate"=TRUE, "Deactivate"=FALSE} ("DER_Control"), "DeviceID"=w288) -> (w285:T7)
          n108 = call "Send Set DER Control Msg.vi"("error in"=w284, "DER_Control"=w285, "SCADA Sub Abstract in"=w286) -> ("error out"=w280:errorcluster, "dup SCADA Sub Abstract"=w283:refnum<class "Blackstart.lvclass">)  [unwired: 7 in]
          n109 = Bundle By Name(cluster=T5 {"DeviceID"="", "Mode"=enum."PQ"} ("DER_setGenerationMode"), "DeviceID"=w288) -> (w279:T5)
          n110 = call "Send Set DER GenerationMode Msg.vi"("error in"=w280, "DER_setGenerationMode"=w279, "SCADA Sub Abstract in"=w283) -> ("error out"=w281:errorcluster, "SCADA Sub Abstract out"=w282:refnum<class "Blackstart.lvclass">)  [unwired: 7 in]
          n111 = Wait (ms)(milliseconds to wait=u32 1000) -> ()  [unwired: 1 out]
        }
        n112 = call "Check for Devices Present.vi"("stop notifier reference"=w264, "error in"=w265, "Devices in"=w263, "Startup Optimization in"=w266) -> ("error out"=w259:errorcluster, "Failed Devices"=w261:T2[], "Startup Optimization out"=w262:refnum<class "Blackstart.lvclass">, "Time has Elapsed"=w260:bool)  [unwired: 4 in]
        n113 = case shown="False" w260 {
          frame False {
            # "Wait for grid to settle"
            n114 = Wait (ms)(milliseconds to wait=u32 1000) -> ()  [unwired: 1 out]
          }
          frame True {
          }
        }
        n115 = Select(t=Blackstart_State."Failure", s=w260, f=Blackstart_State."Success") -> (s? t:f=w276:T1)
      }
      frame "Success" {
        n116 = call "Read Global Configuration.vi"("EMS Generic in"=w297) -> ("Global Configuration"=w296:T8)  [unwired: 8 in, 2 out]
        n117 = Unbundle By Name(w296) -> ("Blackstart Success Wait (sec)"=w295:dbl)
        n118 = Multiply(x=w295, y=1000.0) -> (x*y=w293:dbl)
        n119 = To Unsigned Long Integer(number=w293) -> (unsigned 32bit integer=w292:u32)
        n120 = call "Error Bound Wait (ms).vi"("milliseconds to wait (100)"=w292, "error in"=w306) -> ("error out"=w304:errorcluster)  [unwired: 9 in]
        n121 = call "Send Operation Complete Msg.vi"("error in"=w304, "Operation Complete"=TRUE, "Generic Optimization in"=w297) -> ("error out"=w298:errorcluster, "Generic Optimization out"=w302:refnum<class "Blackstart.lvclass">)  [unwired: 7 in]
        n122 = call "Status Update.vi"("error in"=w298, "Status Update"="Blackstart Successful.") -> ("error out"=w299:errorcluster)  [unwired: 8 in, 1 out]
        n123 = call "Clear Device Groups.vi"("error in"=w299, "Startup Optimization in"=w302) -> ("error out"=w300:errorcluster, "Startup Optimization out"=w301:refnum<class "Blackstart.lvclass">)  [unwired: 8 in]
      }
      frame "Failure", Default {
        n124 = call "Send Operation Complete Msg.vi"("error in"=w316, "Operation Complete"=FALSE ("Activation Complete"), "Generic Optimization in"=w317) -> ("error out"=w312:errorcluster, "Generic Optimization out"=w326:refnum<class "Blackstart.lvclass">)  [unwired: 7 in]
        n125 = Format Into String(format string="Blackstart Failed on %s step." ("Status Update"), w313) -> (resulting string=w319:string, error out=w322:errorcluster)  [unwired: 2 in]
        n126 = Empty Array?(array=w314) -> (empty?=w321:bool)
        n127 = case "Failed Device Array Empty?" shown="False" w321 {
          tunnel: w319 -> [w333 w338]
          tunnel: [w331 w338] -> w320
          tunnel: w314 -> [w335 _]
          tunnel: w322 -> [w330 w337]
          tunnel: [w329 w337] -> w323
          frame False {
            # "Craft failed device message"
            n128 = call <userlib>:"1D Array to String__ogtk.vi"("delimiter (Tab)"=",", "Array of Strings"=w335) -> ("delimited string"=w332:string)  [unwired: 9 in]
            n129 = Format Into String(format string="%s (%s)", error in=w330, w333, w332) -> (resulting string=w331:string, error out=w329:errorcluster)  [unwired: 1 in]
          }
          frame True {
            # "Generic message"
          }
        }
        n130 = call "Status Update.vi"("error in"=w323, "Status Update"=w320) -> ("error out"=w325:errorcluster)  [unwired: 8 in, 1 out]
        n131 = call "Clear Device Groups.vi"("error in"=w325, "Startup Optimization in"=w326) -> ("error out"=w311:errorcluster, "Startup Optimization out"=w315:refnum<class "Blackstart.lvclass">)  [unwired: 8 in]
        n132 = Merge Errors(w312, w311) -> (w310:errorcluster)
      }
    }
    "Status" <- w24
  }
  n133 = call-parent "Actor Core.vi"("error in"=w4, "Actor in"="Blackstart in") -> ("error out"=→"error out":errorcluster, "Actor out"=→"Actor out":refnum<class "Actor.lvclass">)  [unwired: 8 in]
  n134 = flat-sequence {
    tunnel: "Blackstart in" -> [w341]
    frame #0 {
      n135 = call <vilib>:"Read Self Enqueuer.vi"("Actor"=w341) -> ("Self Enqueuer"=w340:refnum<class "Message Enqueuer.lvclass">)  [unwired: 10 in]
      n136 = control-ref of="This VI"() -> (w339:refnum<vi>)
      n137 = call <vilib>:"Send Normal Stop.vi"("Message Enqueuer"=w340) -> ()  [unwired: 10 in, 1 out]
      n138 = invoke class="VI" method="FP.Close"(reference=w339) -> ()  [unwired: 2 in, 3 out]
    }
  }
